vi "Video File Create.vi"(5 "Identifier":string, 6 "Depth Scale (0.001)":dbl=0.001, 7 "Loop? (T)":bool=TRUE, 8 "error in (no error)":errorcluster, 9 "Open File? (T)":bool=TRUE, 10 "Video Path (\"\")":path, 11 "Video File in":refnum<class "Video File.lvclass">) -> (0 "error out":errorcluster, 3 "Video File out":refnum<class "Video File.lvclass">)   [LabVIEW 2018, in "Video File.lvclass"]
uses:
  Video File.lvclass
  Video File.lvclass/Video File.ctl
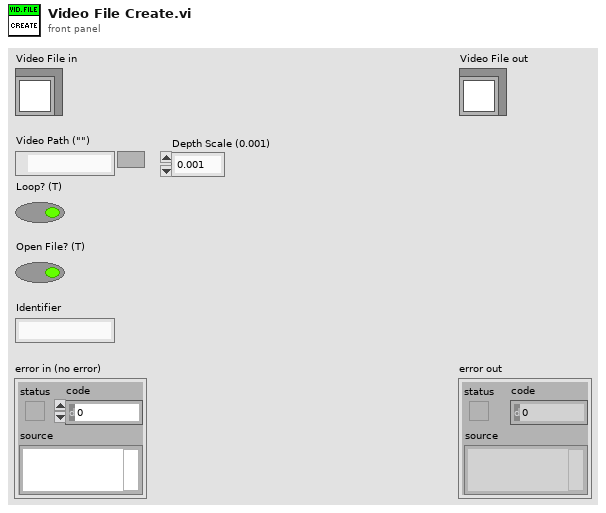
[diagram p1: front panel]
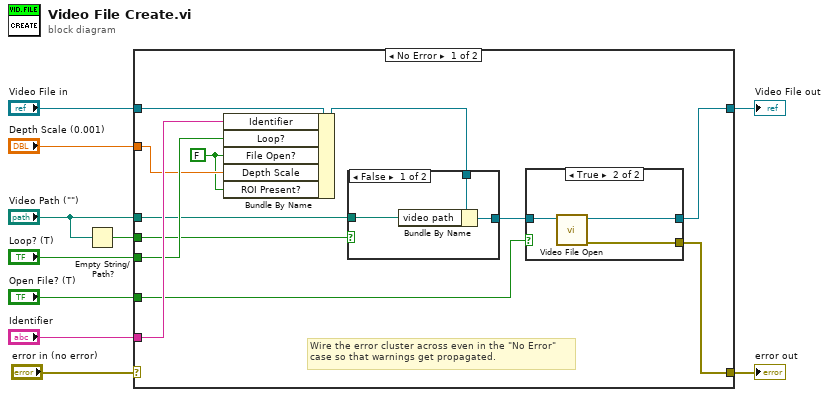
[diagram p0: block diagram]
diagram:
  n1 = Empty String/Path?(string/path="Video Path (\"\")") -> (empty?=w2:bool)
  n2 = case shown="No Error" "error in (no error)" {
    selector: "error in (no error)" -> [_ w32]
    tunnel: [w13 w32] -> w9
    tunnel: [w14 w31] -> w7
    tunnel: "Video File in" -> [w22 w31]
    tunnel: "Video Path (\"\")" -> [w18 _]
    tunnel: "Loop? (T)" -> [w20 _]
    tunnel: "Open File? (T)" -> [w15 _]
    tunnel: "Identifier" -> [w21 _]
    tunnel: w2 -> [w19 _]
    tunnel: "Depth Scale (0.001)" -> [w12 _]
    frame No Error {
      w11 = FALSE ("File Open?")
      # "Wire the error cluster across even in the \"No Error\"\ncase so that warnings get propagated."
      n3 = Bundle By Name(cluster=w22, "Identifier"=w21, "Loop?"=w20, "File Open?"=w11, "Depth Scale"=w12, "ROI Present?"=w11) -> (w17:refnum<class "Video File.lvclass">)
      n4 = case shown="False" w19 {
        tunnel: w18 -> [w28 _]
        tunnel: w17 -> [w29 w30]
        tunnel: [w27 w30] -> w16
        frame False {
          n5 = Bundle By Name(cluster=w29, "video path"=w28) -> (w27:refnum<class "Video File.lvclass">)
        }
        frame True {
        }
      }
      n6 = case shown="True" w15 {
        tunnel: w16 -> [w23 w26]
        tunnel: [w23 w25] -> w14
        tunnel: [_ w24] -> w13
        frame False {
        }
        frame True {
          n7 = call-dynamic "Video File Open.vi"("Video File in"=w26) -> ("error out"=w24:errorcluster, "Video File out"=w25:refnum<class "Video File.lvclass">)  [unwired: 9 in]
        }
      }
    }
    frame Error {
    }
  }
  "error out" <- w9
  "Video File out" <- w7
